vi "Get DDG External Output Step Enabled.vi"(8 "error in (no error)":errorcluster, 10 "puiEnabled":u32, 11 "uiIndex":u32) -> (0 "error out":errorcluster, 2 "puiEnabled out":u32, 3 "function return":u32)   [LabVIEW 2014, in "atmcd32d.lvlib"]
doc: "unsigned int WINAPI GetDDGExternalOutputStepEnabled(at_u32 uiIndex, at_u32 * puiEnabled);"
uses:
  atmcd32d.lvlib
  atmcd32d.dll
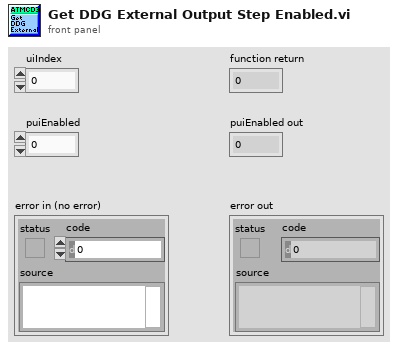
[diagram p1: front panel]
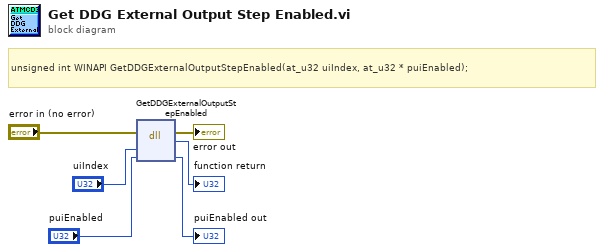
[diagram p0: block diagram]
diagram:
  # "unsigned int WINAPI GetDDGExternalOutputStepEnabled(at_u32 uiIndex, at_u32 * puiEnabled);"
  n1 = dll-call lib="C:/Users/Bakir/Documents/Lambda2-Testing/lib/Andorlib/atmcd32d.*" fn="GetDDGExternalOutputStepEnabled"(error in="error in (no error)", "uiIndex"="uiIndex", "puiEnabled"="puiEnabled") -> (error out=→"error out":errorcluster, →"function return":u32, "puiEnabled"=→"puiEnabled out":u32)  [unwired: 3 in, 1 out]
